vi "transition_count.vi"(4 "previous_state":T2, 6 "current_state":T2, 7 "waitgroup":T1, 8 "error in (no error)":errorcluster, 10 "index in":i32, 11 "recipe_data in":variant) -> (0 "error out":errorcluster, 2 "index out":i32, 3 "recipe_data out":variant)   [LabVIEW 2015, in "example_01.lvlib"]
uses:
  lv-recipe-machine/public/_controls/automatic_state.ctl
  <userlib>/antonio-alexander/lv-waitgroup/public/_controls/api_waitgroup.ctl
  example_01.lvlib
  <userlib>/antonio-alexander/lv-waitgroup/lv-waitgroup.lvlib
  lv-recipe-machine/lv-recipe-machine.lvlib
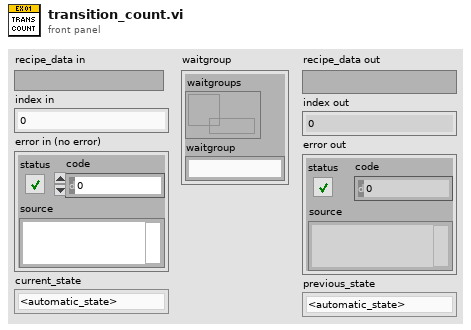
[diagram p1: front panel]
types:
  T1 = typedef "lv-waitgroup.lvlib/api_waitgroup.ctl" = cluster{"waitgroups":refnum<data-value>, "waitgroup":string}
  T2 = typedef "lv-recipe-machine.lvlib/automatic_state.ctl" = enum16{"<automatic_state>", "failed", "idle", "running", "paused", "stopped", "<null>"}
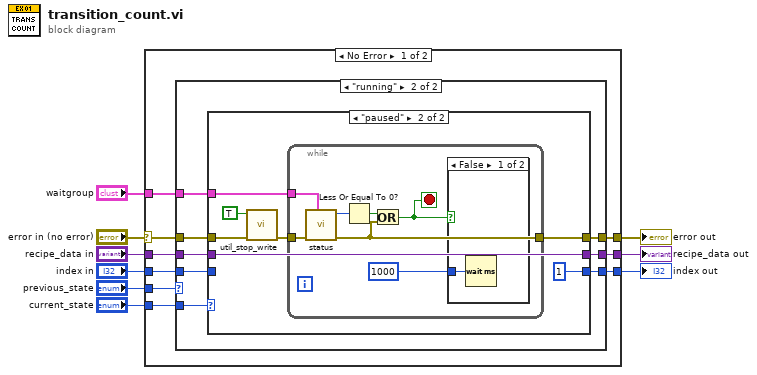
[diagram p0: block diagram]
diagram:
  n1 = case shown="No Error" "error in (no error)" {
    selector: "error in (no error)" -> [w16 w58]
    tunnel: [w15 w58] -> w8
    tunnel: "recipe_data in" -> [w14 w57]
    tunnel: "index in" -> [w12 w56]
    tunnel: "current_state" -> [w17 _]
    tunnel: "previous_state" -> [w18 _]
    tunnel: [w13 w57] -> w3
    tunnel: [w11 w56] -> w2
    tunnel: "waitgroup" -> [w10 _]
    frame No Error {
      n2 = case shown="\"running\"" w18 {
        tunnel: w17 -> [w26 w37]
        tunnel: w16 -> [w22 w33]
        tunnel: [w21 w32] -> w15
        tunnel: w14 -> [w24 w35]
        tunnel: [w23 w34] -> w13
        tunnel: w12 -> [w20 w31]
        tunnel: [w19 w30] -> w11
        tunnel: w10 -> [w25 w36]
        frame Default {
          n3 = case shown="Default" w26 {
            tunnel: w25 -> [_]
            tunnel: w24 -> [w29]
            tunnel: [w29] -> w23
            tunnel: w22 -> [w28]
            tunnel: [w28] -> w21
            tunnel: w20 -> [w27]
            tunnel: [w27] -> w19
            frame Default {
            }
          }
        }
        frame "running" {
          n4 = case shown="\"paused\"" w37 {
            tunnel: w36 -> [_ w43]
            tunnel: w35 -> [w40 w47]
            tunnel: [w40 w47] -> w34
            tunnel: w33 -> [w39 w45]
            tunnel: [w39 w42] -> w32
            tunnel: w31 -> [w38 _]
            tunnel: [w38 1 ("index in")] -> w30
            frame Default {
            }
            frame "paused" {
              n5 = call "util_stop_write.vi"("error in (no error)"=w45, "stop"=TRUE) -> ("error out"=w44:errorcluster)  [unwired: 9 in]
              n6 = while {
                tunnel: w44 -> [w51]
                tunnel: w43 -> [w53]
                tunnel: [w54] -> w42
                stop <- w49 stop-if-true
                n7 = call <userlib>:"status.vi"("waitgroup"=w53, "error in (no error)"=w51) -> ("error out"=w54:errorcluster, "active"=w52:i32)  [unwired: 8 in]
                n8 = Less Or Equal To 0?(x=w52) -> (x <= 0?=w50:bool)
                n9 = Or(x=w50, y=w54) -> (x .or. y?=w49:bool)
                n10 = case shown="False" w49 {
                  tunnel: u32 1000 -> [w55 _]
                  frame False {
                    n11 = Wait (ms)(milliseconds to wait=w55) -> ()  [unwired: 1 out]
                  }
                  frame True {
                  }
                }
              }
            }
          }
        }
      }
    }
    frame Error {
    }
  }
  "error out" <- w8
  "recipe_data out" <- w3
  "index out" <- w2
